vi "Exercise introduction.vi"(5 "Exercise Execution Mode":T1, 6 "Numero USP":dbl format="%#.13f", 7 "Exercise Number":T6, 8 "error in":errorcluster, 9 "Waveform In":waveform(dbl), 10 "Array":bool[](array[boolean]), 11 "Exercise Folder Path":path) -> (0 "error out":errorcluster, 1 "Waveform Out":waveform(dbl), 2 "Done":dbl, 3 "path":path)   [LabVIEW 2014]
uses:
  Ctls/t3q1.ctl
  Ctls/t3q2.ctl
  Ctls/teval.ctl
  Ctls/ExerciseNumeration.ctl
  Ctls/ExerciseState.ctl
  <vilib>/Utility/miscctls.llb/LVPointTypeDef.ctl
  Ctls/radiobutton010.ctl
panel:
  out "Exercise Tab":T2(tab)
  in  "Help?":bool
  in  "TEVAL":T3={"Tamanho"=enum."1", "Tempo Utilizado"=enum."1", "Conteúdo Adequado"=enum."1", "Conteúdo Claro / Coeso"=enum."1", "Adequação à proposta de Reforço das Aulas de Laboratório e de Ensino de LabVIEW"=enum."1", "Contexto dos Problemas Sugeridos"=enum."1", "Contexto das Ferramentas Apresentadas"=enum."1", "Ajuda na compreensão de outras matérias"=enum."1", "compreensão de programação em LabVIEW"=enum."1", "compreensão da teoria apresentada"=enum."1", "compreensão das problemáticas de Instrumentação Elétrica"=enum."1"} caption="Perguntas"
  in  "Close 3":bool
  in  "Close":bool
  in  "T3E1":T4={"F1"=2.0, "F2"=0.0, "F3"=2.0, "A1 (V)"=0.0, "A2 (V)"=0.0, "A3 (V)"=0.0, "A1 (dB)"=0.0, "A2 (dB)"=0.0, "A3 (dB)"=0.0, "Frequência de Corte\nInferior"=0.0, "Ordem do \nFiltro"=0.0} caption="Perguntas:"
  in  "Help? 2":bool
  in  "T3E2":T5
  in  "Close 2":bool
  in  "Help? 3":bool
  # "PSI3214\nLaboratório de Instrumentação Elétrica"
  # "Avaliação do Tutorial"
  # "Ao longo do tutorial foram utilizados materiais em PDF para referência do aluno, materiais em vídeo para acompanhamento mais dinâmico. Neste questionário serão avaliados alguns parâmetros quantitativos a fim de se melhorar a qualidade dos tutoriais fornecidos ao longo dos anos. É importante deixar claro que não será pedida nenhuma informação que possa identificar o aluno, de modo a preservar a privacidade de cada um."
  # "AA.1) Em relação ao Material Escrito disponibilizado em PDF, avalie:"
  # "Muito Pequeno"
  # "Muito Grande"
  # "Pouco Tempo"
  # "Muito Tempo"
  # "Conteúdo do tutorial\npouco adequado às aulas"
  # "Conteúdo do tutorial\nbem adequado às aulas"
  # "Conteúdo do tutorial\nfoi pouco claro/coeso"
  # "Conteúdo do tutorial\nfoi bem claro/coeso"
  # "Tutorial atuou muito mal\ncomo reforço das aulas"
  # "Tutorial atuou muito bem \ncomo reforço das aulas"
  # "Problemas pouco\ncontextualizados"
  # "Problemas muito bem\ncontextualizados"
  # "Ferramentas pouco\ncontextualizadas"
  # "Ferramentas muito bem\ncontextualizadas"
  # "Foi de pouca ajuda na compreensão\nde outras materias"
  # "Foi de grande ajuda na compreensão\nde outras materias"
  # "AA.3) Em relação ao sua compreensão do tutorial, realize uma auto-avaliação sobre sua:"
  # "não compreendi nenhum tópico\nde programação apresentada"
  # "compreendi completamente\ntoda programação apresentada"
  # "não compreendi nenhum tópico\nde teoria apresentada"
  # "compreendi completamente\ntoda teoria apresentada"
  # "não compreendi nenhuma das\nproblemáticas apresentadas"
  # "compreendi completamente\ntodas as problemáticas apresentadas"
  # "PSI3214\nLaboratório de Instrumentação Elétrica"
  # "Exercício 3.1"
  # "Vimos ao longo do tutorial que um filtro é um bloco construtivo que permite a atenuação de certas frequências que compõe nosso sinal. A descrição que foi utilizada até agora se preocupava exclusivamente com as frequências de corte e os tipos de filtro apresentados. Para maioria dos problemas, no entanto, essa descrição é incompleta. Neste exercício veremos outro aspecto de filtros que é muito importante, sua Ordem."
  # "Obs: As escalas dos \neixos X são logarítmicas"
  # "Fig. 1 (a) - Sinal de Entrada"
  # "Fig. 1 (b) - Filtro Butterwoth de Ordem 1"
  # "Veja o exemplo acima, Fig. 1 (a). Na frequência Fa encontra-se nosso sinal de interesse, enquanto que na frequência Fb se encontra um ruído ou uma perturbação, elemento indesejável para análise de nosso sinal. Para que possamos realizar uma construção adequada de nosso filtro devemos, inicialmente, avaliar 3 parâmetros fundamentais: Frequência de Corte, Frequência de Rejeição, Atenuação.\n\n- A Frequência de Corte é definida como o ponto, em nosso filtro, em que a amplitude de nosso sinal cai de 3dB, mas em nosso exemplo inicial vamos escolher a frequência de corte igual à nossa frequência do sinal de interesse, Fa.\n- A Frequência de Rejeição é um ponto de referência, que em conjunto com a Atenuação, define a inclinação da reta r. A inclinação da reta r, por sua vez, varia em passos discretos e possui uma relação íntima com a Ordem de um filtro. De modo geral, um filtro de Ordem 1 possui uma inclinação de -20dB/dec; um filtro de Ordem 2 possui uma inclinação de -40dB/dec; e a cada ordem acrescentada em nosso filtro, adicionamos -20dB/dec em nossa inclinação."
  # "Fig. 2 (a) - Ordem vs Inclinação"
  # "Fig. 2 (b) - Filtro Butterwoth de Ordem 2"
  # "Perceba que a vantagem de se utilizar filtros de Ordem maior se encontra na comparação entre as figuras 1(b) e 2(b). Para uma mesma Frequência de Corte e uma mesma Frequência de Rejeição, conseguimos uma maior atenuação utilizando um filtro de Ordem maior. \n\n    A princípio nos parece óbvia que a utilização de filtros de Ordem Superior é sempre benéfica em um circuito. Contudo são inúmeras as desvantagens da utilização de filtros de Ordens elevadas, as quais não serão tratadas neste tutorial. \n\n    Vamos agora aplicar os conhecimentos estabelecidos acima com um exemplo. Suponha que você se depare com um sinal com as seguintes características:"
  # "Eq. 1 - Equação da Inclinação da Reta r"
  # "Para projetarmos o filtro desejado, deveremos calcular a inclinação da reta r (Mr), que nos dirá qual a inclinação mínima para que sejam cumpridas as especificações desejadas.  Idealmente gostariamos que não houvesse nennhuma mudança entre a amplitude do sinal original e sua amplitude após o filtro, ou seja o ganho deverá ser 1. Por este motivo, escolheremos Fa como a Frequência de Corte. Como queremos atuar na perturbação/ruído que ocorre em Fb, será escolhido Fb como nossa Frequência de Rejeição. A Atenuação na Frequência de Rejeição é arbitrária e será escolhida de acordo com outros requisitos de seu projeto, mas para este exemplo, será escolhida uma atenuação de 50x (ou um ganho de 0.02). Será utilizada a equação Eq. 1 para cálculo da inclinação Mr :"
  # "Deste modo, por meio do calculo da inclinação da reta r sabemos que um filtro de 2 ordem com uma inclinação de -40dB/dec não será suficiente, e que, portanto, deveremos utilizar um filtro de ordem 4, com inclinação de -80dB/dec. Caso façamos as contas invertidas, verificaremos que: para um filtro de ordem 4, teremos um nível de 7.56mV na frequência de rejeição; enquanto que com um filtro de ordem 3, teremos 34,5mV."
  # "Fig. 3 - Resposta do Sinal após Filtragem"
  # "Utilize o VI do exercicio para realizar medições no sinal e reponda:"
  # "Para fechar a tela do enunciado, pressione o botão \"Close Form\""
  # "A) Quais as 3 primeiras frequências dominantes do sinal? Quais suas amplitudes em V e em dB? (Faça uso do maior número de digitos significativos para cálculo das amplitudes)"
  # "Lembre-se: A[dB] = 20.log(A[V])"
  # "B) Considere que queremos filtrar o sinal de modo a que a terceira frequência dominante seja atenuada em 100x. Dê as especificações do filtro passa-baixa a ser utilizado:"
  # "PSI3214\nLaboratório de Instrumentação Elétrica"
  # "Exercício 3.2"
  # "Até o presente momento foram vistos os blocos básicos de construção de um sistema de aquisição de dados. Ao longo dos ultimos 2 tutoriais viu-se a natureza de um conversor AD, a importância de uma etapa de condicionamento do sinal e quais as funcionalidades de um filtro. Vamos agora reunir todos os conceitos vistos para que possamos criar um sistema de aquisição adequado:"
  # "Tomando o diagrama de blocos acima como um guia temos as seguintes etapas de projeto:\n \n1) Analisar quais as características temporais e espectrais que definem a entrada que desejamos adquirir, tais como: níveis de tensão mínimo e máximo e frequências de interesse.\n\n2) Definidas as frequências de interesse, podemos selecionar um ADC com taxa de aquisição adequada (em geral 10x maior do que a maior das frequências de interesse). Em um mesmo momento devemos definir qual a resolução do conversor, dados: uma tensão de fundo de escala (em geral fornecida); uma variação mínima em V do sinal que gostariamos de medir.\n\n3) Com o ADC em mãos, podemos determinar qual o circuito de condicionamento que será utilizado, definindo primeiramente qual sua amplificação, e após isso, qual o Offset DC do sinal. \n\n4) Construído o condicionamento de sinal, podemos finalmente selecionar qual tipo de filtragem será utilizada, definindo a Frequência de Corte, Frequência de Rejeição e a Atenuação desejada na Frequência de Rejeição e, com isso, calculando a ordem do filtro.\n\nTodo o processo descrito acima, na realidade, é muito mais complexo. Contudo, iremos trabalhar com um modelo simplificado para criar uma intuição sobre o processo de aquisição de dados. Vamos utilizar o exercício abaixo para esclarescer quaisquer dúvidas"
  # "Sensor de Pressão Diferencial"
  # "Modifique as configurações do ADC e do Filtro para os valores calculados, e veja como fica o sinal após o processo de conversão  \n\nPara fechar a tela do enunciado, pressione o botão \"Close Form\""
  # "Em uma empresa de engenharia aeronáutica, decidiu-se que você será responsável pela criação de um sistema de aquisição de dados de pressão diferencial para análise estrutural do avião em voo. O sensor de pressão utilizado pela companhia (ilustrado ao lado) é, na realidade, um extensômetro que muda sua resistência com base na deflexão. No gráfico indicado na janela principal do exercício, foram colhidas algumas amostras de dados brutos do sinal, que servirão de base para construção de um sistema de aquisição."
  # "A) Descreva o sinal a ser adquirido, indicando:"
  # "- Níveis de Tensão Globais Máximo e Mínimo:"
  # "- Níveis das três maiores frequências dominantes que compõem o sinal:\n          (Faça uso do maior número de digitos significativos para cálculo das amplitudes)"
  # "Por meio da criação, simulação de modelos do avião e das condições atmosféricas esperadas durante um voo, sabemos que quaisquer variações do sinal do sensor acima de 500 Hz são, na verdade, perturbações espúrias, as quais deverão ser filtradas e retiradas do sinal. Sendo assim, a taxa de aquisição do ADC deverá ser cerca de dez vezes a maior das frequências abaixo de 500Hz.\n    Pelo fato do projeto de um sistema de aquisição de dados estar vinculado a outros sistemas eletrônicos do avião, somos obrigados a utilizar um fundo de escala para o ADC com as tensões V- = 0V e V+=12V. Sabemos que a menor variação do sinal, após a etapa de condicionamento, é de 1mV, logo o LSB do conversor AD deverá ser menor do que esse valor."
  # "B) Selecione as características mais relevantes para o ADC de modo a indicar:"
  # "Como descrito acima, nosso conversor é capaz somente de identificar sinais cujos níveis de tensão estejam dentro do intervalo [0V, 12V]. Sendo assim, gostaríamos que nosso sinal de entrada fosse condicionado para preencher esse intervalo ao máximo."
  # "C) Selecione qual a amplificação e o offset dado pelo circuito de condicionamento de modo a que o sinal ocupe todo o intervalo de medição do conversor AD. Indique:"
  # "Como etapa final do projeto, queremos definir a frequência de rejeição, e sua atenuação correspondente. Assuma que a frequência acima de 500Hz do seu sinal será definida como a frequência de rejeição do filtro. Como o limite de sensibilidade do ADC é de aproximadamente 1mV (dado pelo LSB do conversor), iremos, arbitrariamente, difinir uma atenuação do sinal na frequência de rejeição de 100 vezes, de modo a que não sejam percebidas pelo conversor."
  # "D) Selecione as características do filtro pré-conversor:"
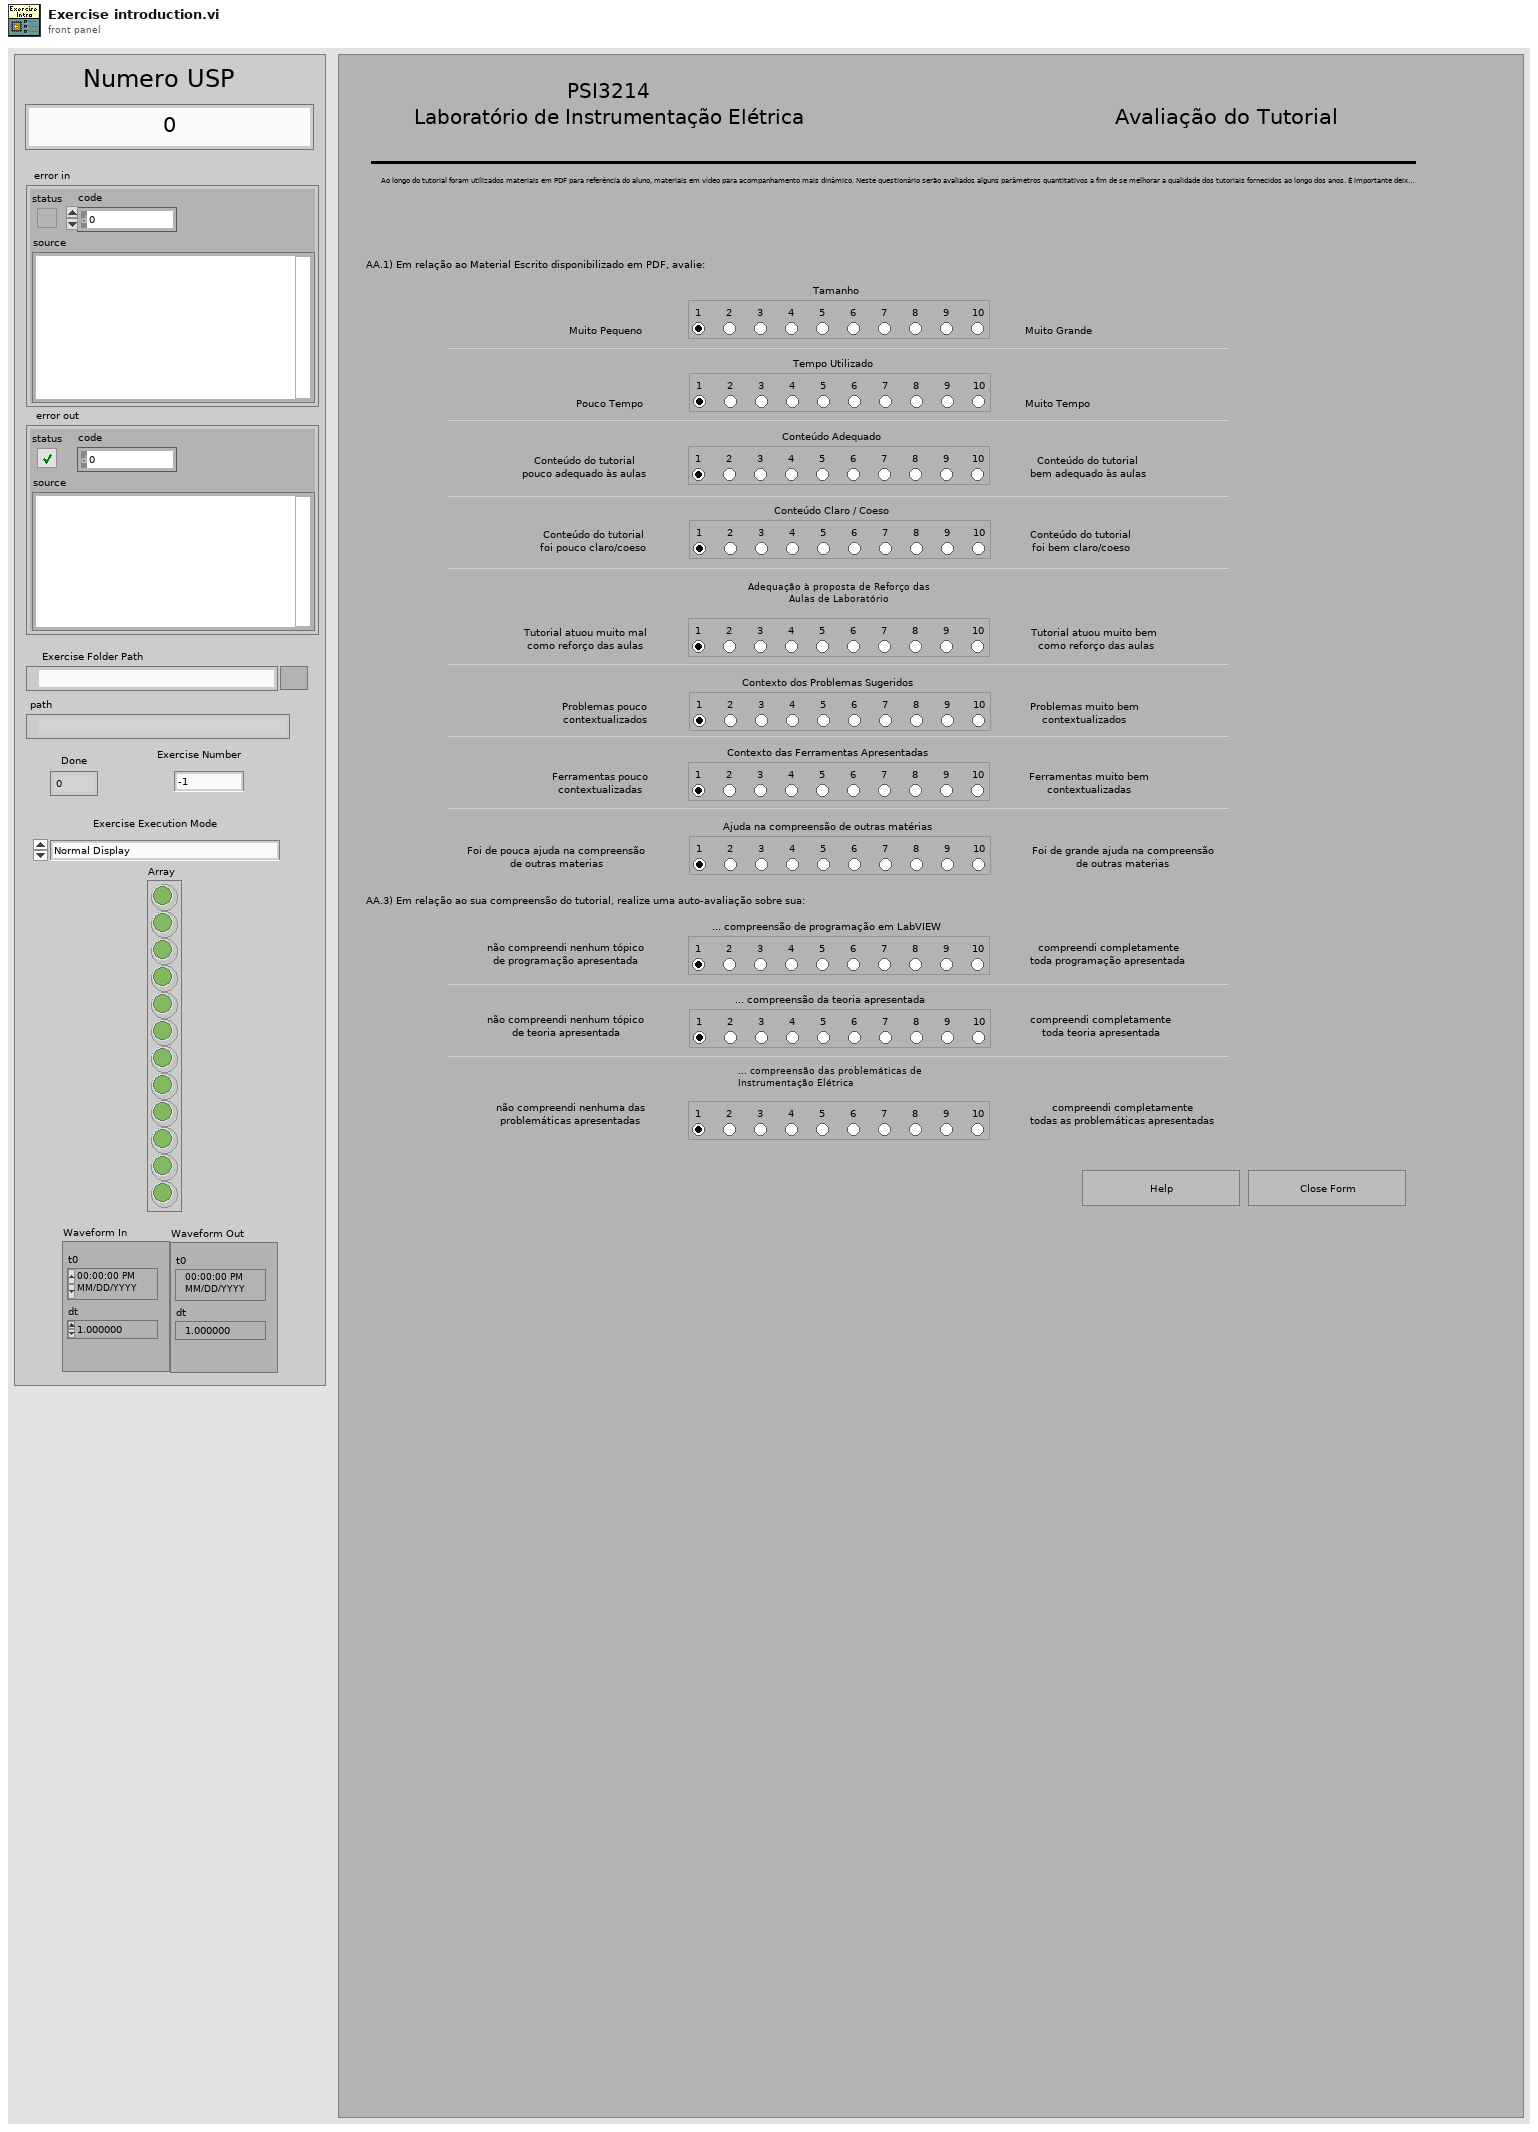
[diagram p1: front panel]
types:
  T1 = typedef "ExerciseState.ctl" = enum16{"Normal Display", "Answer Highligh"}
  T2 = enum32{"Tutorial Evaluation", "Exercicio 1", "Exercicio 2", "Exercício 3", "Exercício 4", "Exercício 5"}
  T3 = typedef "teval.ctl" = cluster{"Tamanho":enum32{"No Selection", "2", "1", "3", "4", "5", "6", "7", "8", "9", "10"}, "Tempo Utilizado":enum32{"No Selection", "2", "1", "3", "4", "5", "6", "7", "8", "9", "10"}, "Conteúdo Adequado":enum32{"No Selection", "2", "1", "3", "4", "5", "6", "7", "8", "9", "10"}, "Conteúdo Claro / Coeso":enum32{"No Selection", "2", "1", "3", "4", "5", "6", "7", "8", "9", "10"}, "Adequação à proposta de Reforço das Aulas de Laboratório e de Ensino de LabVIEW":enum32{"No Selection", "2", "1", "3", "4", "5", "6", "7", "8", "9", "10"}, "Contexto dos Problemas Sugeridos":enum32{"No Selection", "2", "1", "3", "4", "5", "6", "7", "8", "9", "10"}, "Contexto das Ferramentas Apresentadas":enum32{"No Selection", "2", "1", "3", "4", "5", "6", "7", "8", "9", "10"}, "Ajuda na compreensão de outras matérias":enum32{"No Selection", "2", "1", "3", "4", "5", "6", "7", "8", "9", "10"}, "compreensão de programação em LabVIEW":enum32{"No Selection", "2", "1", "3", "4", "5", "6", "7", "8", "9", "10"}, "compreensão da teoria apresentada":enum32{"No Selection", "2", "1", "3", "4", "5", "6", "7", "8", "9", "10"}, "compreensão das problemáticas de Instrumentação Elétrica":enum32{"No Selection", "2", "1", "3", "4", "5", "6", "7", "8", "9", "10"}}
  T4 = typedef "t3q1.ctl" = cluster{"F1":dbl, "F2":dbl, "F3":dbl, "A1 (V)":dbl, "A2 (V)":dbl, "A3 (V)":dbl, "A1 (dB)":dbl, "A2 (dB)":dbl, "A3 (dB)":dbl, "Frequência de Corte\nInferior":dbl, "Ordem do \nFiltro":dbl}
  T5 = typedef "t3q2.ctl" = cluster{"F1 (Hz)":dbl, "F2 (Hz)":dbl, "F3 (Hz)":dbl, "A1 (V)":dbl, "A2 (V)":dbl, "A3 (V)":dbl, "A1 (dB)":dbl, "A2 (dB)":dbl, "A3 (dB)":dbl, "Vmax (V)":dbl, "Vmin (V)":dbl, "Taxa de Aquisição (Hz)":dbl, "Resolução (bits)":dbl, "Offset (V)":dbl, "Amplificação (V/V)":dbl, "Frequência de Corte Inferior (Hz)":dbl, "Ordem do Filtro":dbl}
  T6 = typedef "ExerciseNumeration.ctl" = enum16{"-1", "0", "1", "2", "3", "4", "5", "6", "7", "8", "9", "10"}
  T7 = typedef "LVPointTypeDef.ctl" = cluster{"Horizontal":i16, "Vertical":i16}
  T8 = enum16{"Always On", "Always Off", "Off While Running"}
  T9 = enum16{"open", "replace", "create", "open or create", "replace or create", "replace or create with confirmation"}
  T10 = typedef "radiobutton010.ctl" = enum32{"No Selection", "2", "1", "3", "4", "5", "6", "7", "8", "9", "10"}
  T11 = enum32{"No Selection", "2", "1", "3", "4", "5", "6", "7", "8", "9", "10"}
  T12 = enum32{"No Selection", "2", "1", "3", "4", "5", "6", "7", "8", "9", "10"}[]
  T13 = typedef "imagedata.ctl" = cluster{"image type":i32, "image depth":i32, "image":u8[], "mask":u8[], "colors":u32[], "Rectangle":cluster{"left":i16, "top":i16, "right":i16, "bottom":i16}}
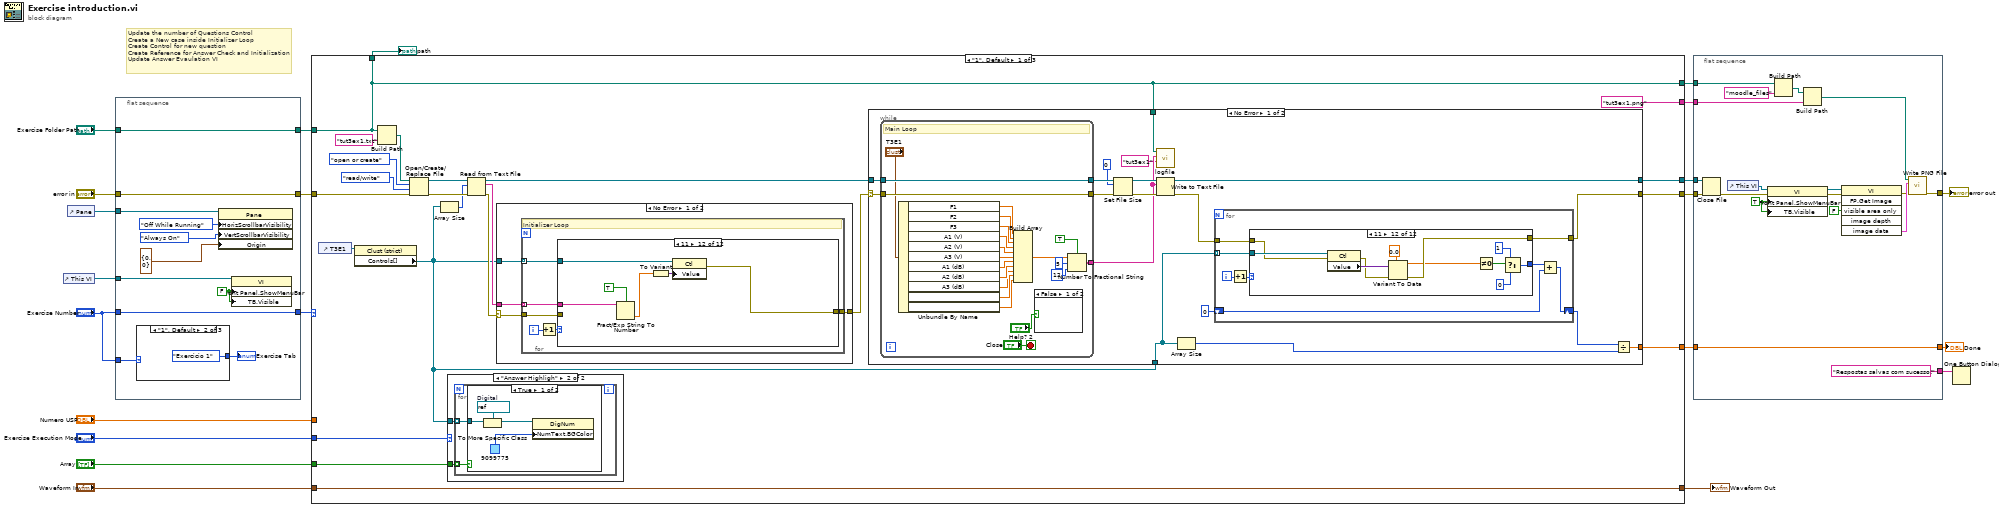
[diagram p0: block diagram]
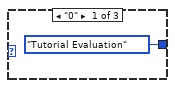
[diagram p2: hidden frame]
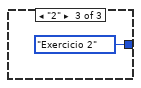
[diagram p3: hidden frame]
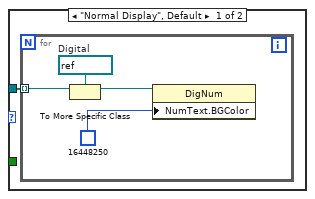
[diagram p4: hidden frame]
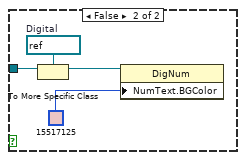
[diagram p5: hidden frame]
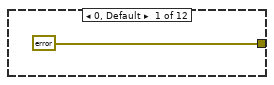
[diagram p6: hidden frame]
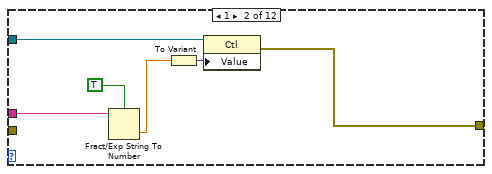
[diagram p7: hidden frame]
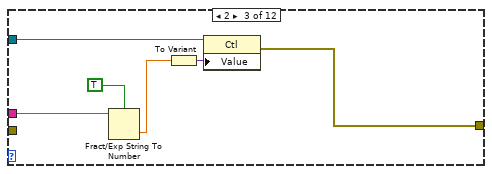
[diagram p8: hidden frame]
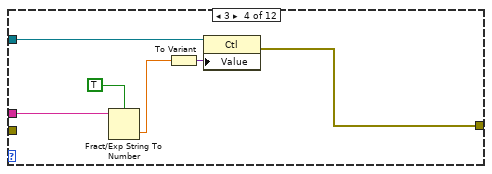
[diagram p9: hidden frame]
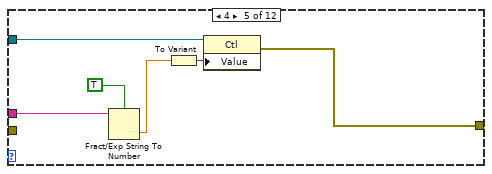
[diagram p10: hidden frame]
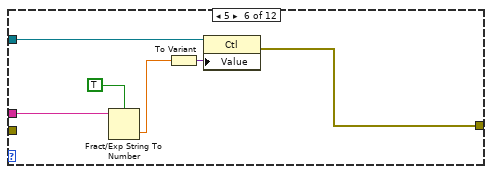
[diagram p11: hidden frame]
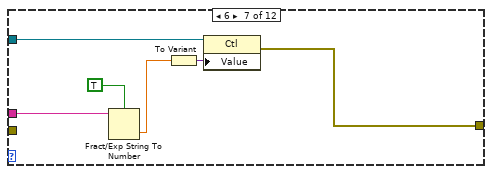
[diagram p12: hidden frame]
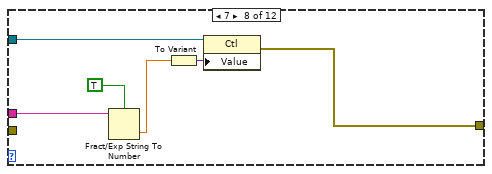
[diagram p13: hidden frame]
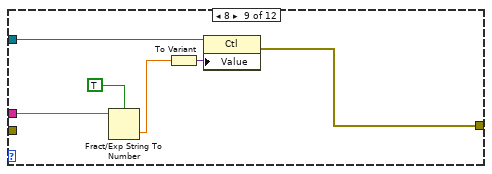
[diagram p14: hidden frame]
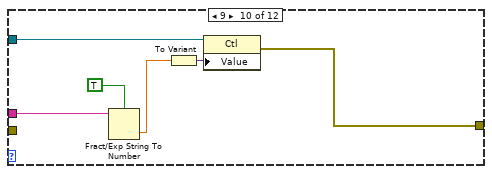
[diagram p15: hidden frame]
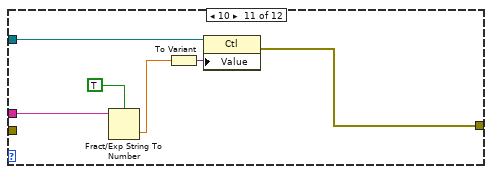
[diagram p16: hidden frame]
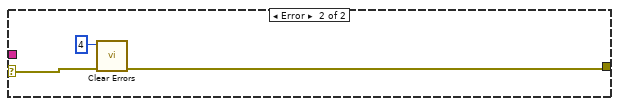
[diagram p17: hidden frame]
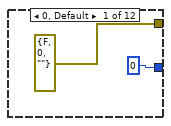
[diagram p18: hidden frame]
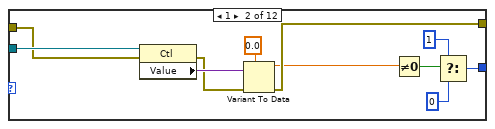
[diagram p19: hidden frame]
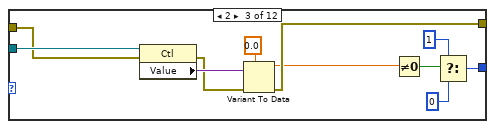
[diagram p20: hidden frame]
diagram:
  # "Update the number of Questions Control\nCreate a New case inside Initializer Loop\nCreate Control for new question\nCreate Reference for Answer Check and Initialization\nUpdate Answer Evaulation VI"
  n1 = control-ref of="This VI"() -> (w20:refnum<vi>)
  n2 = control-ref of="Pane"() -> (w9:refnum<vi>)
  n3 = flat-sequence {
    tunnel: "Exercise Number" -> [w33]
    tunnel: w9 -> [w32]
    tunnel: w20 -> [w31]
    tunnel: "error in" -> [w27]
    tunnel: [w27] -> w18
    tunnel: "Exercise Folder Path" -> [w30]
    tunnel: [w30] -> w16
    tunnel: "Exercise Number" -> [w26]
    tunnel: [w26] -> w14
    frame #0 {
      w29 = FALSE ("Front Panel Window:Show Menu Bar")
      n4 = case shown="\"1\", Default" w33 {
        tunnel: [T2."Tutorial Evaluation" ("Exercise Tab") T2."Exercicio 1" ("Exercise Tab") T2."Exercicio 2" ("Exercise Tab")] -> w24
        frame "0" {
        }
        frame "1", Default {
        }
        frame "2" {
        }
      }
      "Exercise Tab" <- w24
      n5 = property class="Pane"(reference=w32, "HorizScrollbarVisibility"=T8."Off While Running" ("Horizontal Scrollbar Visibility"), "VertScrollbarVisibility"=T8."Always On" ("Vertical Scrollbar Visibility"), "Origin"=T7 {"Horizontal"=0, "Vertical"=0}) -> ()  [unwired: 1 in, 2 out]
      n6 = property class="VI"(reference=w31, "Front Panel.ShowMenuBar"=w29, "TB.Visible"=w29) -> ()  [unwired: 1 in, 2 out]
    }
  }
  n7 = case shown="\"1\", Default" w14 {
    tunnel: w16 -> [w38 w330 w729]
    tunnel: w18 -> [w56 w348 w745]
    tunnel: [w50 w342 w739] -> w22
    tunnel: [w49 w341 w738] -> w21
    tunnel: [w45 w337 w734] -> w11
    tunnel: [w38 w330 w729] -> w10
    tunnel: "Array" -> [w39 w332 _]
    tunnel: "Exercise Execution Mode" -> [w40 w333 _]
    tunnel: "Waveform In" -> [w42 w334 w730]
    tunnel: [w42 w334 w730] -> w5
    tunnel: [w38 w330 w729] -> w3
    tunnel: ["tut3ex1.png" ("name or relative path") "tut3ex2.png" ("name or relative path") "tut3eval.png" ("name or relative path")] -> w2
    tunnel: "Numero USP" -> [_ _ _]
    frame "1", Default {
      n8 = control-ref of="T3E1"() -> (w43:refnum<vi>)
      n9 = property class="Clust (strict)"(reference=w43) -> ("Controls[]"=w41:refnum<vi>[])  [unwired: 1 in, 2 out]
      n10 = Build Path(base path=w38, name or relative path="tut3ex1.txt") -> (appended path=w57:path)
      n11 = Open/Create/Replace File(file path (use dialog)=w57, error in=w56, operation (0:open)=T9."open or create", access (0:read/write)=enum16{"read/write", "read-only", "write-only"}."read/write") -> (refnum out=w53:refnum<file>, error out=w52:errorcluster)  [unwired: 2 in, 1 out]
      n12 = Array Size(array=w41) -> (size(s)=w44:i32)
      n13 = case shown="\"Answer Highligh\"" w40 {
        tunnel: w41 -> [w59 w65]
        tunnel: w39 -> [_ w64]
        frame "Normal Display", Default {
          n14 = for {
            tunnel: w59 -> [w63] mode=indexing
            w61 = refnum<vi> refnum  # Digital
            n15 = To More Specific Class(target class=w61, reference=w63) -> (specific class reference=w62:refnum<vi>)  [unwired: 1 in, 1 out]
            n16 = property class="DigNum"(reference=w62, "NumText.BGColor"=u32 16448250) -> ()  [unwired: 1 in, 2 out]
          }
        }
        frame "Answer Highligh" {
          n17 = for {
            tunnel: w65 -> [w67] mode=indexing
            tunnel: w64 -> [w66] mode=indexing
            n18 = case shown="True" w66 {
              tunnel: w67 -> [w70 w75]
              frame True {
                w68 = refnum<vi> refnum  # Digital
                n19 = To More Specific Class(target class=w68, reference=w70) -> (specific class reference=w69:refnum<vi>)  [unwired: 1 in, 1 out]
                n20 = property class="DigNum"(reference=w69, "NumText.BGColor"=u32 9099775) -> ()  [unwired: 1 in, 2 out]
              }
              frame False {
                w73 = refnum<vi> refnum  # Digital
                n21 = To More Specific Class(target class=w73, reference=w75) -> (specific class reference=w74:refnum<vi>)  [unwired: 1 in, 1 out]
                n22 = property class="DigNum"(reference=w74, "NumText.BGColor"=u32 15517125) -> ()  [unwired: 1 in, 2 out]
              }
            }
          }
        }
      }
      n23 = Read from Text File(file (use dialog)=w53, count=w44, error in=w52) -> (refnum out=w51:refnum<file>, text=w47:string[], error out=w48:errorcluster)  [unwired: 1 in, 1 out]
      n24 = case shown="No Error" w48 {
        selector: w48 -> [w78 w155]
        tunnel: w47 -> [w79 _]
        tunnel: [w77 w154] -> w46
        tunnel: w41 -> [w76 _]
        frame No Error {
          n25 = for {
            tunnel: w79 -> [w85] mode=indexing
            tunnel: [w82] -> w77
            tunnel: w78 -> [w81]
            tunnel: w76 -> [w80] mode=indexing
            i -> [w83]
            # "Initializer Loop"
            n26 = Increment(x=w83) -> (x+1=w84:i32)
            n27 = case shown="11" w84 {
              tunnel: w85 -> [_ w90 w96 w102 w108 w114 w120 w126 w132 w138 w144 w150]
              tunnel: [errorcluster {"status"=FALSE, "code"=0, "source"=""} ("error out") w92 w98 w104 w110 w116 w122 w128 w134 w140 w146 w152] -> w82
              tunnel: w81 -> [_ _ _ _ _ _ _ _ _ _ _ _]
              tunnel: w80 -> [_ w91 w97 w103 w109 w115 w121 w127 w133 w139 w145 w151]
              frame 0, Default {
              }
              frame 1 {
                n28 = Fract/Exp String To Number(use system decimal point (T)=TRUE, string=w90) -> (number=w88:dbl)  [unwired: 2 in, 1 out]
                n29 = To Variant(anything=w88) -> (Variant=w89:variant)
                n30 = property class="Ctl"(reference=w91, "Value"=w89) -> (error out=w92:errorcluster)  [unwired: 1 in, 1 out]
              }
              frame 2 {
                n31 = Fract/Exp String To Number(use system decimal point (T)=TRUE, string=w96) -> (number=w94:dbl)  [unwired: 2 in, 1 out]
                n32 = To Variant(anything=w94) -> (Variant=w95:variant)
                n33 = property class="Ctl"(reference=w97, "Value"=w95) -> (error out=w98:errorcluster)  [unwired: 1 in, 1 out]
              }
              frame 3 {
                n34 = Fract/Exp String To Number(use system decimal point (T)=TRUE, string=w102) -> (number=w100:dbl)  [unwired: 2 in, 1 out]
                n35 = To Variant(anything=w100) -> (Variant=w101:variant)
                n36 = property class="Ctl"(reference=w103, "Value"=w101) -> (error out=w104:errorcluster)  [unwired: 1 in, 1 out]
              }
              frame 4 {
                n37 = Fract/Exp String To Number(use system decimal point (T)=TRUE, string=w108) -> (number=w106:dbl)  [unwired: 2 in, 1 out]
                n38 = To Variant(anything=w106) -> (Variant=w107:variant)
                n39 = property class="Ctl"(reference=w109, "Value"=w107) -> (error out=w110:errorcluster)  [unwired: 1 in, 1 out]
              }
              frame 5 {
                n40 = Fract/Exp String To Number(use system decimal point (T)=TRUE, string=w114) -> (number=w112:dbl)  [unwired: 2 in, 1 out]
                n41 = To Variant(anything=w112) -> (Variant=w113:variant)
                n42 = property class="Ctl"(reference=w115, "Value"=w113) -> (error out=w116:errorcluster)  [unwired: 1 in, 1 out]
              }
              frame 6 {
                n43 = Fract/Exp String To Number(use system decimal point (T)=TRUE, string=w120) -> (number=w118:dbl)  [unwired: 2 in, 1 out]
                n44 = To Variant(anything=w118) -> (Variant=w119:variant)
                n45 = property class="Ctl"(reference=w121, "Value"=w119) -> (error out=w122:errorcluster)  [unwired: 1 in, 1 out]
              }
              frame 7 {
                n46 = Fract/Exp String To Number(use system decimal point (T)=TRUE, string=w126) -> (number=w124:dbl)  [unwired: 2 in, 1 out]
                n47 = To Variant(anything=w124) -> (Variant=w125:variant)
                n48 = property class="Ctl"(reference=w127, "Value"=w125) -> (error out=w128:errorcluster)  [unwired: 1 in, 1 out]
              }
              frame 8 {
                n49 = Fract/Exp String To Number(use system decimal point (T)=TRUE, string=w132) -> (number=w130:dbl)  [unwired: 2 in, 1 out]
                n50 = To Variant(anything=w130) -> (Variant=w131:variant)
                n51 = property class="Ctl"(reference=w133, "Value"=w131) -> (error out=w134:errorcluster)  [unwired: 1 in, 1 out]
              }
              frame 9 {
                n52 = Fract/Exp String To Number(use system decimal point (T)=TRUE, string=w138) -> (number=w136:dbl)  [unwired: 2 in, 1 out]
                n53 = To Variant(anything=w136) -> (Variant=w137:variant)
                n54 = property class="Ctl"(reference=w139, "Value"=w137) -> (error out=w140:errorcluster)  [unwired: 1 in, 1 out]
              }
              frame 10 {
                n55 = Fract/Exp String To Number(use system decimal point (T)=TRUE, string=w144) -> (number=w142:dbl)  [unwired: 2 in, 1 out]
                n56 = To Variant(anything=w142) -> (Variant=w143:variant)
                n57 = property class="Ctl"(reference=w145, "Value"=w143) -> (error out=w146:errorcluster)  [unwired: 1 in, 1 out]
              }
              frame 11 {
                n58 = Fract/Exp String To Number(use system decimal point (T)=TRUE, string=w150) -> (number=w148:dbl)  [unwired: 2 in, 1 out]
                n59 = To Variant(anything=w148) -> (Variant=w149:variant)
                n60 = property class="Ctl"(reference=w151, "Value"=w149) -> (error out=w152:errorcluster)  [unwired: 1 in, 1 out]
              }
            }
          }
        }
        frame Error {
          n61 = call <vilib>:"Clear Errors.vi"("error in (no error)"=w155, "specific error code to clear (0: all)"=4) -> ("error out"=w154:errorcluster)  [unwired: 4 in, 1 out]
        }
      }
      n62 = case shown="No Error" w46 {
        selector: w46 -> [w172 w327]
        tunnel: w51 -> [w173 w328]
        tunnel: [w160 w327] -> w50
        tunnel: [w171 w328] -> w49
        tunnel: [w164 -1.0] -> w45
        tunnel: w41 -> [w163 _]
        tunnel: w38 -> [w157 _]
        frame No Error {
          n63 = while {
            tunnel: w173 -> [w324]
            tunnel: w172 -> [w323]
            tunnel: [w324] -> w168
            tunnel: [w323] -> w170
            tunnel: [w313] -> w158
            stop <- "Close" stop-if-true
            # "Main Loop"
            n64 = Unbundle By Name("T3E1") -> ("F1"=w307:dbl, "F2"=w308:dbl, "F3"=w322:dbl, "A1 (V)"=w321:dbl, "A2 (V)"=w320:dbl, "A3 (V)"=w319:dbl, "A1 (dB)"=w318:dbl, "A2 (dB)"=w317:dbl, "A3 (dB)"=w316:dbl, "Frequência de Corte\nInferior"=w315:dbl, "Ordem do \nFiltro"=w314:dbl)
            n65 = Build Array(w307, w308, w322, w321, w320, w319, w318, w317, w316, w315, w314) -> (w312:dbl[])
            n66 = case shown="False" "Help? 2" {
              frame False {
              }
              frame True {
                n67 = call "Greteer.vi"() -> ()  [unwired: 10 in, 2 out]
              }
            }
            n68 = Number To Fractional String(use system decimal point (T)=TRUE, number=w312, width (-)=i16 5, precision (6)=i16 12) -> (F-format string=w313:string[])
          }
          n69 = Set File Size(4:w170, 6:i64 0 ("size (in bytes)"), 7:w168) -> (0:w169:errorcluster, 3:w167:refnum<file>)
          n70 = call "logfile.vi"("from"="tut3ex1", "Text In"=w158, "Path In"=w157) -> ()  [unwired: 7 in, 2 out]
          n71 = Write to Text File(file (use dialog)=w167, text=w158, error in=w169) -> (refnum out=w171:refnum<file>, error out=w161:errorcluster)  [unwired: 1 in, 1 out]
          n72 = Array Size(array=w163) -> (size(s)=w162:i32)
          n73 = for {
            shift-right: [w178] -> w165
            shift-left: 0 -> [w177]
            tunnel: w163 -> [w176] mode=indexing
            tunnel: w161 -> [w175]
            tunnel: [w174] -> w160
            i -> [w180]
            n74 = Increment(x=w180) -> (x+1=w181:i32)
            n75 = case shown="11" w181 {
              tunnel: [0 ("f") w192 w203 w214 w225 w236 w247 w258 w269 w280 w291 w302] -> w179
              tunnel: w176 -> [_ w189 w200 w211 w222 w233 w244 w255 w266 w277 w288 w299]
              tunnel: w175 -> [_ w188 w199 w210 w221 w232 w243 w254 w265 w276 w287 w298]
              tunnel: [errorcluster {"status"=FALSE, "code"=0, "source"=""} ("error out") w186 w197 w208 w219 w230 w241 w252 w263 w274 w285 w296] -> w174
              frame 0, Default {
              }
              frame 1 {
                n76 = property class="Ctl"(reference=w189, error in=w188) -> (error out=w187:errorcluster, "Value"=w190:variant)  [unwired: 1 out]
                n77 = Variant To Data(error in=w187, type=0.0 ("y"), Variant=w190) -> (data=w184:dbl, error out=w186:errorcluster)
                n78 = Not Equal To 0?(x=w184) -> (x != 0?=w185:bool)
                n79 = Select(t=1, s=w185, f=0) -> (s? t:f=w192:i32)
              }
              frame 2 {
                n80 = property class="Ctl"(reference=w200, error in=w199) -> (error out=w198:errorcluster, "Value"=w201:variant)  [unwired: 1 out]
                n81 = Variant To Data(error in=w198, type=0.0 ("y"), Variant=w201) -> (data=w195:dbl, error out=w197:errorcluster)
                n82 = Not Equal To 0?(x=w195) -> (x != 0?=w196:bool)
                n83 = Select(t=1, s=w196, f=0) -> (s? t:f=w203:i32)
              }
              frame 3 {
                n84 = property class="Ctl"(reference=w211, error in=w210) -> (error out=w209:errorcluster, "Value"=w212:variant)  [unwired: 1 out]
                n85 = Variant To Data(error in=w209, type=0.0 ("y"), Variant=w212) -> (data=w206:dbl, error out=w208:errorcluster)
                n86 = Not Equal To 0?(x=w206) -> (x != 0?=w207:bool)
                n87 = Select(t=1, s=w207, f=0) -> (s? t:f=w214:i32)
              }
              frame 4 {
                n88 = property class="Ctl"(reference=w222, error in=w221) -> (error out=w220:errorcluster, "Value"=w223:variant)  [unwired: 1 out]
                n89 = Variant To Data(error in=w220, type=0.0 ("y"), Variant=w223) -> (data=w217:dbl, error out=w219:errorcluster)
                n90 = Not Equal To 0?(x=w217) -> (x != 0?=w218:bool)
                n91 = Select(t=1, s=w218, f=0) -> (s? t:f=w225:i32)
              }
              frame 5 {
                n92 = property class="Ctl"(reference=w233, error in=w232) -> (error out=w231:errorcluster, "Value"=w234:variant)  [unwired: 1 out]
                n93 = Variant To Data(error in=w231, type=0.0 ("y"), Variant=w234) -> (data=w228:dbl, error out=w230:errorcluster)
                n94 = Not Equal To 0?(x=w228) -> (x != 0?=w229:bool)
                n95 = Select(t=1, s=w229, f=0) -> (s? t:f=w236:i32)
              }
              frame 6 {
                n96 = property class="Ctl"(reference=w244, error in=w243) -> (error out=w242:errorcluster, "Value"=w245:variant)  [unwired: 1 out]
                n97 = Variant To Data(error in=w242, type=0.0 ("y"), Variant=w245) -> (data=w239:dbl, error out=w241:errorcluster)
                n98 = Not Equal To 0?(x=w239) -> (x != 0?=w240:bool)
                n99 = Select(t=1, s=w240, f=0) -> (s? t:f=w247:i32)
              }
              frame 7 {
                n100 = property class="Ctl"(reference=w255, error in=w254) -> (error out=w253:errorcluster, "Value"=w256:variant)  [unwired: 1 out]
                n101 = Variant To Data(error in=w253, type=0.0 ("y"), Variant=w256) -> (data=w250:dbl, error out=w252:errorcluster)
                n102 = Not Equal To 0?(x=w250) -> (x != 0?=w251:bool)
                n103 = Select(t=1, s=w251, f=0) -> (s? t:f=w258:i32)
              }
              frame 8 {
                n104 = property class="Ctl"(reference=w266, error in=w265) -> (error out=w264:errorcluster, "Value"=w267:variant)  [unwired: 1 out]
                n105 = Variant To Data(error in=w264, type=0.0 ("y"), Variant=w267) -> (data=w261:dbl, error out=w263:errorcluster)
                n106 = Not Equal To 0?(x=w261) -> (x != 0?=w262:bool)
                n107 = Select(t=1, s=w262, f=0) -> (s? t:f=w269:i32)
              }
              frame 9 {
                n108 = property class="Ctl"(reference=w277, error in=w276) -> (error out=w275:errorcluster, "Value"=w278:variant)  [unwired: 1 out]
                n109 = Variant To Data(error in=w275, type=0.0 ("y"), Variant=w278) -> (data=w272:dbl, error out=w274:errorcluster)
                n110 = Not Equal To 0?(x=w272) -> (x != 0?=w273:bool)
                n111 = Select(t=1, s=w273, f=0) -> (s? t:f=w280:i32)
              }
              frame 10 {
                n112 = property class="Ctl"(reference=w288, error in=w287) -> (error out=w286:errorcluster, "Value"=w289:variant)  [unwired: 1 out]
                n113 = Variant To Data(error in=w286, type=0.0 ("y"), Variant=w289) -> (data=w283:dbl, error out=w285:errorcluster)
                n114 = Not Equal To 0?(x=w283) -> (x != 0?=w284:bool)
                n115 = Select(t=1, s=w284, f=0) -> (s? t:f=w291:i32)
              }
              frame 11 {
                n116 = property class="Ctl"(reference=w299, error in=w298) -> (error out=w297:errorcluster, "Value"=w300:variant)  [unwired: 1 out]
                n117 = Variant To Data(error in=w297, type=0.0 ("y"), Variant=w300) -> (data=w294:dbl, error out=w296:errorcluster)
                n118 = Not Equal To 0?(x=w294) -> (x != 0?=w295:bool)
                n119 = Select(t=1, s=w295, f=0) -> (s? t:f=w302:i32)
              }
            }
            n120 = Add(x=w179, y=w177) -> (x+y=w178:i32)
          }
          n121 = Divide(x=w165, y=w162) -> (x/y=w164:dbl)
        }
        frame Error {
        }
      }
    }
    frame "2" {
      n122 = control-ref of="T3E2"() -> (w335:refnum<vi>)
      n123 = property class="Clust (strict)"(reference=w335) -> ("Controls[]"=w331:refnum<vi>[])  [unwired: 1 in, 2 out]
      n124 = Build Path(base path=w330, name or relative path="tut3ex2.txt") -> (appended path=w349:path)
      n125 = Open/Create/Replace File(file path (use dialog)=w349, error in=w348, operation (0:open)=T9."open or create", access (0:read/write)=enum16{"read/write", "read-only", "write-only"}."read/write") -> (refnum out=w345:refnum<file>, error out=w344:errorcluster)  [unwired: 2 in, 1 out]
      n126 = case shown="\"Answer Highligh\"" w333 {
        tunnel: w331 -> [w351 w357]
        tunnel: w332 -> [_ w356]
        frame "Normal Display", Default {
          n127 = for {
            tunnel: w351 -> [w355] mode=indexing
            w353 = refnum<vi> refnum  # Digital
            n128 = To More Specific Class(target class=w353, reference=w355) -> (specific class reference=w354:refnum<vi>)  [unwired: 1 in, 1 out]
            n129 = property class="DigNum"(reference=w354, "NumText.BGColor"=u32 16448250) -> ()  [unwired: 1 in, 2 out]
          }
        }
        frame "Answer Highligh" {
          n130 = for {
            tunnel: w357 -> [w359] mode=indexing
            tunnel: w356 -> [w358] mode=indexing
            n131 = case shown="True" w358 {
              tunnel: w359 -> [w362 w367]
              frame True {
                w360 = refnum<vi> refnum  # Digital
                n132 = To More Specific Class(target class=w360, reference=w362) -> (specific class reference=w361:refnum<vi>)  [unwired: 1 in, 1 out]
                n133 = property class="DigNum"(reference=w361, "NumText.BGColor"=u32 9099775) -> ()  [unwired: 1 in, 2 out]
              }
              frame False {
                w365 = refnum<vi> refnum  # Digital
                n134 = To More Specific Class(target class=w365, reference=w367) -> (specific class reference=w366:refnum<vi>)  [unwired: 1 in, 1 out]
                n135 = property class="DigNum"(reference=w366, "NumText.BGColor"=u32 15517125) -> ()  [unwired: 1 in, 2 out]
              }
            }
          }
        }
      }
      n136 = Array Size(array=w331) -> (size(s)=w336:i32)
      n137 = Read from Text File(file (use dialog)=w345, count=w336, error in=w344) -> (refnum out=w343:refnum<file>, text=w339:string[], error out=w340:errorcluster)  [unwired: 1 in, 1 out]
      n138 = case shown="No Error" w340 {
        selector: w340 -> [w370 w483]
        tunnel: w339 -> [w371 _]
        tunnel: [w369 w482] -> w338
        tunnel: w331 -> [w368 _]
        frame No Error {
          n139 = for {
            tunnel: w371 -> [w374] mode=indexing
            tunnel: [w372] -> w369
            tunnel: w370 -> [w375]
            tunnel: w368 -> [w373] mode=indexing
            i -> [w377]
            # "Initializer Loop"
            n140 = Increment(x=w377) -> (x+1=w376:i32)
            n141 = case shown="17" w376 {
              tunnel: w374 -> [_ w382 w388 w394 w400 w406 w412 w418 w424 w430 w436 w442 w448 w454 w460 w466 w472 w478]
              tunnel: [errorcluster {"status"=FALSE, "code"=0, "source"=""} ("error out") w384 w390 w396 w402 w408 w414 w420 w426 w432 w438 w444 w450 w456 w462 w468 w474 w480] -> w372
              tunnel: w373 -> [_ w383 w389 w395 w401 w407 w413 w419 w425 w431 w437 w443 w449 w455 w461 w467 w473 w479]
              tunnel: w375 -> [_ _ _ _ _ _ _ _ _ _ _ _ _ _ _ _ _ _]
              frame 0, Default {
              }
              frame 1 {
                n142 = Fract/Exp String To Number(use system decimal point (T)=TRUE, string=w382) -> (number=w380:dbl)  [unwired: 2 in, 1 out]
                n143 = To Variant(anything=w380) -> (Variant=w381:variant)
                n144 = property class="Ctl"(reference=w383, "Value"=w381) -> (error out=w384:errorcluster)  [unwired: 1 in, 1 out]
              }
              frame 2 {
                n145 = Fract/Exp String To Number(use system decimal point (T)=TRUE, string=w388) -> (number=w386:dbl)  [unwired: 2 in, 1 out]
                n146 = To Variant(anything=w386) -> (Variant=w387:variant)
                n147 = property class="Ctl"(reference=w389, "Value"=w387) -> (error out=w390:errorcluster)  [unwired: 1 in, 1 out]
              }
              frame 3 {
                n148 = Fract/Exp String To Number(use system decimal point (T)=TRUE, string=w394) -> (number=w392:dbl)  [unwired: 2 in, 1 out]
                n149 = To Variant(anything=w392) -> (Variant=w393:variant)
                n150 = property class="Ctl"(reference=w395, "Value"=w393) -> (error out=w396:errorcluster)  [unwired: 1 in, 1 out]
              }
              frame 4 {
                n151 = Fract/Exp String To Number(use system decimal point (T)=TRUE, string=w400) -> (number=w398:dbl)  [unwired: 2 in, 1 out]
                n152 = To Variant(anything=w398) -> (Variant=w399:variant)
                n153 = property class="Ctl"(reference=w401, "Value"=w399) -> (error out=w402:errorcluster)  [unwired: 1 in, 1 out]
              }
              frame 5 {
                n154 = Fract/Exp String To Number(use system decimal point (T)=TRUE, string=w406) -> (number=w404:dbl)  [unwired: 2 in, 1 out]
                n155 = To Variant(anything=w404) -> (Variant=w405:variant)
                n156 = property class="Ctl"(reference=w407, "Value"=w405) -> (error out=w408:errorcluster)  [unwired: 1 in, 1 out]
              }
              frame 6 {
                n157 = Fract/Exp String To Number(use system decimal point (T)=TRUE, string=w412) -> (number=w410:dbl)  [unwired: 2 in, 1 out]
                n158 = To Variant(anything=w410) -> (Variant=w411:variant)
                n159 = property class="Ctl"(reference=w413, "Value"=w411) -> (error out=w414:errorcluster)  [unwired: 1 in, 1 out]
              }
              frame 7 {
                n160 = Fract/Exp String To Number(use system decimal point (T)=TRUE, string=w418) -> (number=w416:dbl)  [unwired: 2 in, 1 out]
                n161 = To Variant(anything=w416) -> (Variant=w417:variant)
                n162 = property class="Ctl"(reference=w419, "Value"=w417) -> (error out=w420:errorcluster)  [unwired: 1 in, 1 out]
              }
              frame 8 {
                n163 = Fract/Exp String To Number(use system decimal point (T)=TRUE, string=w424) -> (number=w422:dbl)  [unwired: 2 in, 1 out]
                n164 = To Variant(anything=w422) -> (Variant=w423:variant)
                n165 = property class="Ctl"(reference=w425, "Value"=w423) -> (error out=w426:errorcluster)  [unwired: 1 in, 1 out]
              }
              frame 9 {
                n166 = Fract/Exp String To Number(use system decimal point (T)=TRUE, string=w430) -> (number=w428:dbl)  [unwired: 2 in, 1 out]
                n167 = To Variant(anything=w428) -> (Variant=w429:variant)
                n168 = property class="Ctl"(reference=w431, "Value"=w429) -> (error out=w432:errorcluster)  [unwired: 1 in, 1 out]
              }
              frame 10 {
                n169 = Fract/Exp String To Number(use system decimal point (T)=TRUE, string=w436) -> (number=w434:dbl)  [unwired: 2 in, 1 out]
                n170 = To Variant(anything=w434) -> (Variant=w435:variant)
                n171 = property class="Ctl"(reference=w437, "Value"=w435) -> (error out=w438:errorcluster)  [unwired: 1 in, 1 out]
              }
              frame 11 {
                n172 = Fract/Exp String To Number(use system decimal point (T)=TRUE, string=w442) -> (number=w440:dbl)  [unwired: 2 in, 1 out]
                n173 = To Variant(anything=w440) -> (Variant=w441:variant)
                n174 = property class="Ctl"(reference=w443, "Value"=w441) -> (error out=w444:errorcluster)  [unwired: 1 in, 1 out]
              }
              frame 12 {
                n175 = Fract/Exp String To Number(use system decimal point (T)=TRUE, string=w448) -> (number=w446:dbl)  [unwired: 2 in, 1 out]
                n176 = To Variant(anything=w446) -> (Variant=w447:variant)
                n177 = property class="Ctl"(reference=w449, "Value"=w447) -> (error out=w450:errorcluster)  [unwired: 1 in, 1 out]
              }
              frame 13 {
                n178 = Fract/Exp String To Number(use system decimal point (T)=TRUE, string=w454) -> (number=w452:dbl)  [unwired: 2 in, 1 out]
                n179 = To Variant(anything=w452) -> (Variant=w453:variant)
                n180 = property class="Ctl"(reference=w455, "Value"=w453) -> (error out=w456:errorcluster)  [unwired: 1 in, 1 out]
              }
              frame 14 {
                n181 = Fract/Exp String To Number(use system decimal point (T)=TRUE, string=w460) -> (number=w458:dbl)  [unwired: 2 in, 1 out]
                n182 = To Variant(anything=w458) -> (Variant=w459:variant)
                n183 = property class="Ctl"(reference=w461, "Value"=w459) -> (error out=w462:errorcluster)  [unwired: 1 in, 1 out]
              }
              frame 15 {
                n184 = Fract/Exp String To Number(use system decimal point (T)=TRUE, string=w466) -> (number=w464:dbl)  [unwired: 2 in, 1 out]
                n185 = To Variant(anything=w464) -> (Variant=w465:variant)
                n186 = property class="Ctl"(reference=w467, "Value"=w465) -> (error out=w468:errorcluster)  [unwired: 1 in, 1 out]
              }
              frame 16 {
                n187 = Fract/Exp String To Number(use system decimal point (T)=TRUE, string=w472) -> (number=w470:dbl)  [unwired: 2 in, 1 out]
                n188 = To Variant(anything=w470) -> (Variant=w471:variant)
                n189 = property class="Ctl"(reference=w473, "Value"=w471) -> (error out=w474:errorcluster)  [unwired: 1 in, 1 out]
              }
              frame 17 {
                n190 = Fract/Exp String To Number(use system decimal point (T)=TRUE, string=w478) -> (number=w476:dbl)  [unwired: 2 in, 1 out]
                n191 = To Variant(anything=w476) -> (Variant=w477:variant)
                n192 = property class="Ctl"(reference=w479, "Value"=w477) -> (error out=w480:errorcluster)  [unwired: 1 in, 1 out]
              }
            }
          }
        }
        frame Error {
          n193 = call <vilib>:"Clear Errors.vi"("error in (no error)"=w483, "specific error code to clear (0: all)"=4) -> ("error out"=w482:errorcluster)  [unwired: 4 in, 1 out]
        }
      }
      n194 = case shown="No Error" w338 {
        selector: w338 -> [w499 w726]
        tunnel: w343 -> [w500 w727]
        tunnel: [w487 w726] -> w342
        tunnel: [w498 w727] -> w341
        tunnel: [w491 -1.0] -> w337
        tunnel: w331 -> [w490 _]
        tunnel: w330 -> [w485 _]
        frame No Error {
          n195 = while {
            tunnel: w500 -> [w724]
            tunnel: w499 -> [w723]
            tunnel: [w724] -> w495
            tunnel: [w723] -> w497
            tunnel: [w700] -> w486
            stop <- "Close 2" stop-if-true
            # "Main Loop"
            n196 = Unbundle By Name("T3E2") -> ("F1 (Hz)"=w720:dbl, "F2 (Hz)"=w719:dbl, "F3 (Hz)"=w718:dbl, "A1 (V)"=w717:dbl, "A2 (V)"=w716:dbl, "A3 (V)"=w715:dbl, "A1 (dB)"=w714:dbl, "A2 (dB)"=w713:dbl, "A3 (dB)"=w712:dbl, "Vmax (V)"=w711:dbl, "Vmin (V)"=w710:dbl, "Taxa de Aquisição (Hz)"=w709:dbl, "Resolução (bits)"=w708:dbl, "Offset (V)"=w707:dbl, "Amplificação (V/V)"=w706:dbl, "Frequência de Corte Inferior (Hz)"=w705:dbl, "Ordem do Filtro"=w704:dbl)
            n197 = Build Array(w720, w719, w718, w717, w716, w715, w714, w713, w712, w711, w710, w709, w708, w707, w706, w705, w704) -> (w699:dbl[])
            n198 = case shown="True" "Help? 3" {
              frame False {
              }
              frame True {
                n199 = call "Greteer.vi"() -> ()  [unwired: 10 in, 2 out]
              }
            }
            n200 = Number To Fractional String(use system decimal point (T)=TRUE, number=w699, width (-)=i16 5, precision (6)=i16 12) -> (F-format string=w700:string[])
          }
          n201 = Set File Size(4:w497, 6:i64 0 ("size (in bytes)"), 7:w495) -> (0:w496:errorcluster, 3:w494:refnum<file>)
          n202 = Write to Text File(file (use dialog)=w494, text=w486, error in=w496) -> (refnum out=w498:refnum<file>, error out=w488:errorcluster)  [unwired: 1 in, 1 out]
          n203 = call "logfile.vi"("from"="tut3ex2", "Text In"=w486, "Path In"=w485) -> ()  [unwired: 7 in, 2 out]
          n204 = Array Size(array=w490) -> (size(s)=w489:i32)
          n205 = for {
            shift-right: [w507] -> w492
            shift-left: _ -> [w506]
            tunnel: w490 -> [w504] mode=indexing
            tunnel: w488 -> [w503]
            tunnel: [w501] -> w487
            i -> [w508]
            n206 = Increment(x=w508) -> (x+1=w505:i32)
            n207 = case shown="17" w505 {
              tunnel: [0 ("f") w519 w530 w541 w552 w563 w574 w585 w596 w607 w618 w629 w640 w651 w662 w673 w684 w695] -> w502
              tunnel: w504 -> [_ w516 w527 w538 w549 w560 w571 w582 w593 w604 w615 w626 w637 w648 w659 w670 w681 w692]
              tunnel: w503 -> [_ w515 w526 w537 w548 w559 w570 w581 w592 w603 w614 w625 w636 w647 w658 w669 w680 w691]
              tunnel: [errorcluster {"status"=FALSE, "code"=0, "source"=""} ("error out") w513 w524 w535 w546 w557 w568 w579 w590 w601 w612 w623 w634 w645 w656 w667 w678 w689] -> w501
              frame 0, Default {
              }
              frame 1 {
                n208 = property class="Ctl"(reference=w516, error in=w515) -> (error out=w514:errorcluster, "Value"=w517:variant)  [unwired: 1 out]
                n209 = Variant To Data(error in=w514, type=0.0 ("y"), Variant=w517) -> (data=w511:dbl, error out=w513:errorcluster)
                n210 = Not Equal To 0?(x=w511) -> (x != 0?=w512:bool)
                n211 = Select(t=1, s=w512, f=0) -> (s? t:f=w519:i32)
              }
              frame 2 {
                n212 = property class="Ctl"(reference=w527, error in=w526) -> (error out=w525:errorcluster, "Value"=w528:variant)  [unwired: 1 out]
                n213 = Variant To Data(error in=w525, type=0.0 ("y"), Variant=w528) -> (data=w522:dbl, error out=w524:errorcluster)
                n214 = Not Equal To 0?(x=w522) -> (x != 0?=w523:bool)
                n215 = Select(t=1, s=w523, f=0) -> (s? t:f=w530:i32)
              }
              frame 3 {
                n216 = property class="Ctl"(reference=w538, error in=w537) -> (error out=w536:errorcluster, "Value"=w539:variant)  [unwired: 1 out]
                n217 = Variant To Data(error in=w536, type=0.0 ("y"), Variant=w539) -> (data=w533:dbl, error out=w535:errorcluster)
                n218 = Not Equal To 0?(x=w533) -> (x != 0?=w534:bool)
                n219 = Select(t=1, s=w534, f=0) -> (s? t:f=w541:i32)
              }
              frame 4 {
                n220 = property class="Ctl"(reference=w549, error in=w548) -> (error out=w547:errorcluster, "Value"=w550:variant)  [unwired: 1 out]
                n221 = Variant To Data(error in=w547, type=0.0 ("y"), Variant=w550) -> (data=w544:dbl, error out=w546:errorcluster)
                n222 = Not Equal To 0?(x=w544) -> (x != 0?=w545:bool)
                n223 = Select(t=1, s=w545, f=0) -> (s? t:f=w552:i32)
              }
              frame 5 {
                n224 = property class="Ctl"(reference=w560, error in=w559) -> (error out=w558:errorcluster, "Value"=w561:variant)  [unwired: 1 out]
                n225 = Variant To Data(error in=w558, type=0.0 ("y"), Variant=w561) -> (data=w555:dbl, error out=w557:errorcluster)
                n226 = Not Equal To 0?(x=w555) -> (x != 0?=w556:bool)
                n227 = Select(t=1, s=w556, f=0) -> (s? t:f=w563:i32)
              }
              frame 6 {
                n228 = property class="Ctl"(reference=w571, error in=w570) -> (error out=w569:errorcluster, "Value"=w572:variant)  [unwired: 1 out]
                n229 = Variant To Data(error in=w569, type=0.0 ("y"), Variant=w572) -> (data=w566:dbl, error out=w568:errorcluster)
                n230 = Not Equal To 0?(x=w566) -> (x != 0?=w567:bool)
                n231 = Select(t=1, s=w567, f=0) -> (s? t:f=w574:i32)
              }
              frame 7 {
                n232 = property class="Ctl"(reference=w582, error in=w581) -> (error out=w580:errorcluster, "Value"=w583:variant)  [unwired: 1 out]
                n233 = Variant To Data(error in=w580, type=0.0 ("y"), Variant=w583) -> (data=w577:dbl, error out=w579:errorcluster)
                n234 = Not Equal To 0?(x=w577) -> (x != 0?=w578:bool)
                n235 = Select(t=1, s=w578, f=0) -> (s? t:f=w585:i32)
              }
              frame 8 {
                n236 = property class="Ctl"(reference=w593, error in=w592) -> (error out=w591:errorcluster, "Value"=w594:variant)  [unwired: 1 out]
                n237 = Variant To Data(error in=w591, type=0.0 ("y"), Variant=w594) -> (data=w588:dbl, error out=w590:errorcluster)
                n238 = Not Equal To 0?(x=w588) -> (x != 0?=w589:bool)
                n239 = Select(t=1, s=w589, f=0) -> (s? t:f=w596:i32)
              }
              frame 9 {
                n240 = property class="Ctl"(reference=w604, error in=w603) -> (error out=w602:errorcluster, "Value"=w605:variant)  [unwired: 1 out]
                n241 = Variant To Data(error in=w602, type=0.0 ("y"), Variant=w605) -> (data=w599:dbl, error out=w601:errorcluster)
                n242 = Not Equal To 0?(x=w599) -> (x != 0?=w600:bool)
                n243 = Select(t=1, s=w600, f=0) -> (s? t:f=w607:i32)
              }
              frame 10 {
                n244 = property class="Ctl"(reference=w615, error in=w614) -> (error out=w613:errorcluster, "Value"=w616:variant)  [unwired: 1 out]
                n245 = Variant To Data(error in=w613, type=0.0 ("y"), Variant=w616) -> (data=w610:dbl, error out=w612:errorcluster)
                n246 = Not Equal To 0?(x=w610) -> (x != 0?=w611:bool)
                n247 = Select(t=1, s=w611, f=0) -> (s? t:f=w618:i32)
              }
              frame 11 {
                n248 = property class="Ctl"(reference=w626, error in=w625) -> (error out=w624:errorcluster, "Value"=w627:variant)  [unwired: 1 out]
                n249 = Variant To Data(error in=w624, type=0.0 ("y"), Variant=w627) -> (data=w621:dbl, error out=w623:errorcluster)
                n250 = Not Equal To 0?(x=w621) -> (x != 0?=w622:bool)
                n251 = Select(t=1, s=w622, f=0) -> (s? t:f=w629:i32)
              }
              frame 12 {
                n252 = property class="Ctl"(reference=w637, error in=w636) -> (error out=w635:errorcluster, "Value"=w638:variant)  [unwired: 1 out]
                n253 = Variant To Data(error in=w635, type=0.0 ("y"), Variant=w638) -> (data=w632:dbl, error out=w634:errorcluster)
                n254 = Not Equal To 0?(x=w632) -> (x != 0?=w633:bool)
                n255 = Select(t=1, s=w633, f=0) -> (s? t:f=w640:i32)
              }
              frame 13 {
                n256 = property class="Ctl"(reference=w648, error in=w647) -> (error out=w646:errorcluster, "Value"=w649:variant)  [unwired: 1 out]
                n257 = Variant To Data(error in=w646, type=0.0 ("y"), Variant=w649) -> (data=w643:dbl, error out=w645:errorcluster)
                n258 = Not Equal To 0?(x=w643) -> (x != 0?=w644:bool)
                n259 = Select(t=1, s=w644, f=0) -> (s? t:f=w651:i32)
              }
              frame 14 {
                n260 = property class="Ctl"(reference=w659, error in=w658) -> (error out=w657:errorcluster, "Value"=w660:variant)  [unwired: 1 out]
                n261 = Variant To Data(error in=w657, type=0.0 ("y"), Variant=w660) -> (data=w654:dbl, error out=w656:errorcluster)
                n262 = Not Equal To 0?(x=w654) -> (x != 0?=w655:bool)
                n263 = Select(t=1, s=w655, f=0) -> (s? t:f=w662:i32)
              }
              frame 15 {
                n264 = property class="Ctl"(reference=w670, error in=w669) -> (error out=w668:errorcluster, "Value"=w671:variant)  [unwired: 1 out]
                n265 = Variant To Data(error in=w668, type=0.0 ("y"), Variant=w671) -> (data=w665:dbl, error out=w667:errorcluster)
                n266 = Not Equal To 0?(x=w665) -> (x != 0?=w666:bool)
                n267 = Select(t=1, s=w666, f=0) -> (s? t:f=w673:i32)
              }
              frame 16 {
                n268 = property class="Ctl"(reference=w681, error in=w680) -> (error out=w679:errorcluster, "Value"=w682:variant)  [unwired: 1 out]
                n269 = Variant To Data(error in=w679, type=0.0 ("y"), Variant=w682) -> (data=w676:dbl, error out=w678:errorcluster)
                n270 = Not Equal To 0?(x=w676) -> (x != 0?=w677:bool)
                n271 = Select(t=1, s=w677, f=0) -> (s? t:f=w684:i32)
              }
              frame 17 {
                n272 = property class="Ctl"(reference=w692, error in=w691) -> (error out=w690:errorcluster, "Value"=w693:variant)  [unwired: 1 out]
                n273 = Variant To Data(error in=w690, type=0.0 ("y"), Variant=w693) -> (data=w687:dbl, error out=w689:errorcluster)
                n274 = Not Equal To 0?(x=w687) -> (x != 0?=w688:bool)
                n275 = Select(t=1, s=w688, f=0) -> (s? t:f=w695:i32)
              }
            }
            n276 = Add(x=w502, y=w506) -> (x+y=w507:i32)
          }
          n277 = Divide(x=w492, y=w489) -> (x/y=w491:dbl)
        }
        frame Error {
        }
      }
    }
    frame "0" {
      n278 = control-ref of="TEVAL"() -> (w732:refnum<vi>)
      n279 = property class="Clust (strict)"(reference=w732) -> ("Controls[]"=w731:refnum<vi>[])  [unwired: 1 in, 2 out]
      n280 = Build Path(base path=w729, name or relative path="teval.txt") -> (appended path=w746:path)
      n281 = Open/Create/Replace File(file path (use dialog)=w746, error in=w745, operation (0:open)=T9."open or create", access (0:read/write)=enum16{"read/write", "read-only", "write-only"}."read/write") -> (refnum out=w742:refnum<file>, error out=w741:errorcluster)  [unwired: 2 in, 1 out]
      n282 = Array Size(array=w731) -> (size(s)=w733:i32)
      n283 = Read from Text File(file (use dialog)=w742, count=w733, error in=w741) -> (refnum out=w740:refnum<file>, text=w736:string[], error out=w737:errorcluster)  [unwired: 1 in, 1 out]
      n284 = case shown="No Error" w737 {
        selector: w737 -> [w750 w792]
        tunnel: w736 -> [w751 _]
        tunnel: [w749 w791] -> w735
        tunnel: w731 -> [w748 _]
        frame No Error {
          n285 = for {
            tunnel: w751 -> [w761] mode=indexing
            tunnel: [w760] -> w749
            tunnel: w750 -> [w759]
            tunnel: w748 -> [w758] mode=indexing
            # "Initializer Loop"
            n286 = Scan From String(format string="%d", input string=w761, error in=w759) -> (error out=w756:errorcluster, output 1=w754:i32)  [unwired: 2 in, 2 out]
            n287 = To Unsigned Long Integer(number=w754) -> (unsigned 32bit integer=w755:u32)
            n288 = case shown="No Error" w756 {
              selector: w756 -> [w763 w788]
              tunnel: w755 -> [w765 _]
              tunnel: [w764 radiobutton010."2" ("Radio Buttons")] -> w753
              tunnel: [w762 w788] -> w752
              frame No Error {
                n289 = case shown="10" w765 {
                  tunnel: [radiobutton010."No Selection" ("Radio Buttons") radiobutton010."1" ("Radio Buttons") radiobutton010."2" ("Radio Buttons") radiobutton010."3" ("Radio Buttons") radiobutton010."4" ("Radio Buttons") radiobutton010."5" ("Radio Buttons") radiobutton010."6" ("Radio Buttons") radiobutton010."7" ("Radio Buttons") radiobutton010."8" ("Radio Buttons") radiobutton010."9" ("Radio Buttons") radiobutton010."10" ("Radio Buttons")] -> w764
                  tunnel: w763 -> [w766 w769 w771 w773 w775 w777 w779 w781 w783 w785 w787]
                  tunnel: [w766 w769 w771 w773 w775 w777 w779 w781 w783 w785 w787] -> w762
                  frame 0, Default {
                  }
                  frame 1 {
                  }
                  frame 2 {
                  }
                  frame 3 {
                  }
                  frame 4 {
                  }
                  frame 5 {
                  }
                  frame 6 {
                  }
                  frame 7 {
                  }
                  frame 8 {
                  }
                  frame 9 {
                  }
                  frame 10 {
                  }
                }
              }
              frame Error {
              }
            }
            n290 = property class="Ctl"(reference=w758, error in=w752, "Val(Sgnl)"=w753) -> (error out=w760:errorcluster)  [unwired: 1 out]
          }
        }
        frame Error {
          n291 = call <vilib>:"Clear Errors.vi"("error in (no error)"=w792, "specific error code to clear (0: all)"=4) -> ("error out"=w791:errorcluster)  [unwired: 4 in, 1 out]
        }
      }
      n292 = case shown="No Error" w735 {
        selector: w735 -> [w808 w843]
        tunnel: w740 -> [w809 w844]
        tunnel: [w796 w843] -> w739
        tunnel: [w807 w844] -> w738
        tunnel: [w800 -1.0] -> w734
        tunnel: w731 -> [w799 _]
        tunnel: w729 -> [w794 _]
        frame No Error {
          n293 = while {
            tunnel: w809 -> [w841]
            tunnel: w808 -> [w840]
            tunnel: [w841] -> w804
            tunnel: [w840] -> w806
            tunnel: [w825] -> w795
            stop <- "Close 3" stop-if-true
            # "Main Loop"
            n294 = Unbundle By Name("TEVAL") -> ("Tamanho"=w838:T11, "Tempo Utilizado"=w837:T11, "Conteúdo Adequado"=w836:T11, "Conteúdo Claro / Coeso"=w835:T11, "Adequação à proposta de Reforço das Aulas de Laboratório e de Ensino de LabVIEW"=w834:T11, "Contexto dos Problemas Sugeridos"=w833:T11, "Contexto das Ferramentas Apresentadas"=w832:T11, "Ajuda na compreensão de outras matérias"=w831:T11, "compreensão de programação em LabVIEW"=w830:T11, "compreensão da teoria apresentada"=w829:T11, "compreensão das problemáticas de Instrumentação Elétrica"=w828:T11)
            n295 = Build Array(w838, w837, w836, w835, w834, w833, w832, w831, w830, w829, w828) -> (w827:T12)
            n296 = case shown="True" "Help?" {
              frame False {
              }
              frame True {
                n297 = call "Greteer.vi"() -> ()  [unwired: 10 in, 2 out]
              }
            }
            n298 = Number To Decimal String(number=w827, width (-)=i16 2) -> (decimal integer string=w825:string[])
          }
          n299 = Set File Size(4:w806, 6:i64 0 ("size (in bytes)"), 7:w804) -> (0:w805:errorcluster, 3:w803:refnum<file>)
          n300 = call "logfile.vi"("from"="tut3eval", "Text In"=w795, "Path In"=w794) -> ()  [unwired: 7 in, 2 out]
          n301 = Write to Text File(file (use dialog)=w803, text=w795, error in=w805) -> (refnum out=w807:refnum<file>, error out=w797:errorcluster)  [unwired: 1 in, 1 out]
          n302 = for {
            shift-right: [w821] -> w801
            shift-left: _ -> [w820]
            tunnel: w799 -> [w819] mode=indexing
            tunnel: w797 -> [w818]
            tunnel: [w817] -> w796
            w812 = radiobutton010."No Selection" ("y")
            # "Check for Valid Response"
            n303 = property class="Ctl"(reference=w819, error in=w818) -> (error out=w810:errorcluster, "Value"=w813:variant)  [unwired: 1 out]
            n304 = Variant To Data(error in=w810, type=w812, Variant=w813) -> (data=w811:T10, error out=w817:errorcluster)
            n305 = Not Equal?(x=w811, y=w812) -> (x != y?=w816:bool)
            n306 = Select(t=1, s=w816, f=0) -> (s? t:f=w822:i32)
            n307 = Add(x=w822, y=w820) -> (x+y=w821:i32)
          }
          n308 = Array Size(array=w799) -> (size(s)=w798:i32)
          n309 = Divide(x=w801, y=w798) -> (x/y=w800:dbl)
        }
        frame Error {
        }
      }
    }
  }
  "path" <- w10
  "Waveform Out" <- w5
  n310 = flat-sequence {
    tunnel: w22 -> [w862]
    tunnel: w21 -> [w861]
    tunnel: [w848] -> w13
    tunnel: [w857] -> w12
    tunnel: w11 -> [w857]
    tunnel: ["Respostas salvas com sucesso!" ("message")] -> w4
    tunnel: w3 -> [w846]
    tunnel: w2 -> [w855]
    frame #0 {
      w859 = TRUE ("Front Panel Window:Show Menu Bar")
      n311 = Close File(refnum=w861, error in=w862) -> (error out=w858:errorcluster)  [unwired: 1 out]
      n312 = control-ref of="This VI"() -> (w860:refnum<vi>)
      n313 = property class="VI"(reference=w860, error in=w858, "Front Panel.ShowMenuBar"=w859, "TB.Visible"=w859) -> (reference out=w852:refnum<vi>, error out=w851:errorcluster)
      n314 = Build Path(base path=w846, name or relative path="moodle_files") -> (appended path=w847:path)
      n315 = Build Path(base path=w847, name or relative path=w855) -> (appended path=w849:path)
      n316 = invoke class="VI" method="FP.Get Image"(reference=w852, error in=w851, "visible area only"=FALSE ("Visible Area Only")) -> (error out=w850:errorcluster, "image data"=w854:T13)  [unwired: 3 in, 4 out]
      n317 = call <vilib>:"Write PNG File.vi"("error in (no error)"=w850, "image data"=w854, "path to PNG file"=w849) -> ("error out"=w848:errorcluster)  [unwired: 7 in, 1 out]
    }
  }
  n318 = One Button Dialog(message=w4) -> ()  [unwired: 1 in, 1 out]
  "error out" <- w13
  "Done" <- w12
